vi "Disconnect.vi"(0 "reference in":refnum<class "SwitchBase.lvclass">, 1 "channel 1":string caption="Chan", 5 "error in (no error)":errorcluster) -> (14 "reference in":refnum<class "SwitchBase.lvclass">, 19 "error out":errorcluster)   [LabVIEW 2017]
uses:
  SwitchBase.lvclass
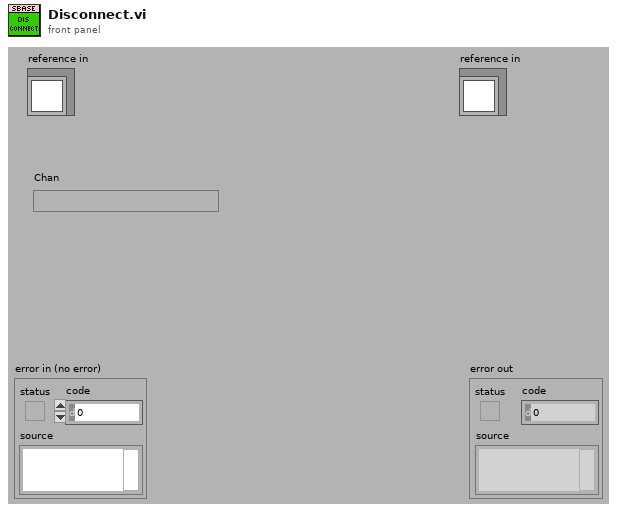
[diagram p1: front panel]
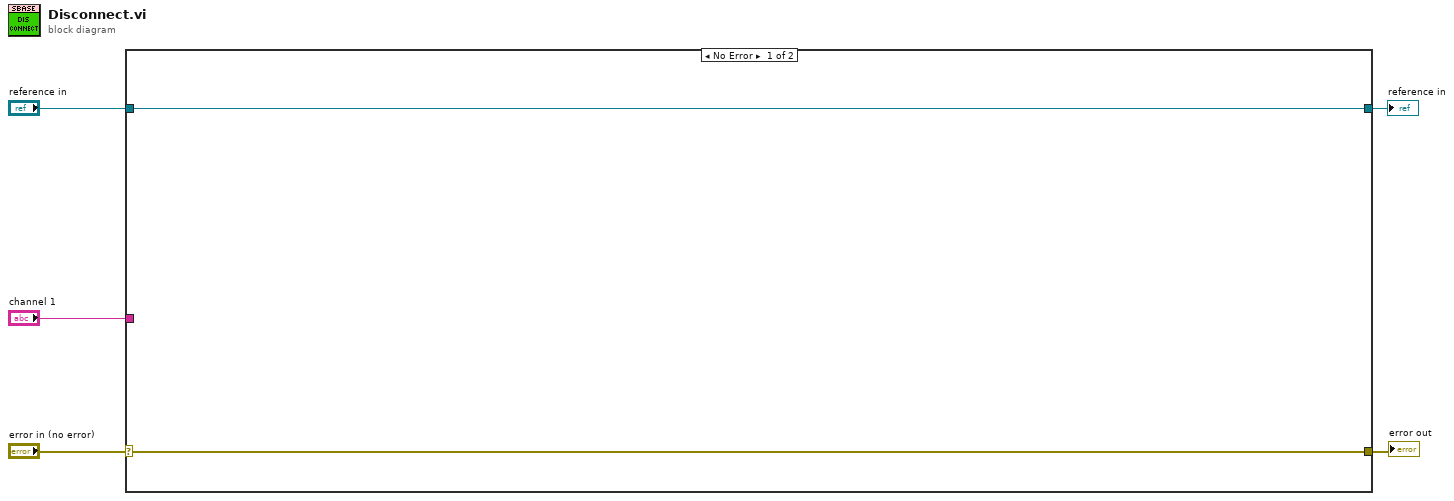
[diagram p0: block diagram]
diagram:
  n1 = case shown="No Error" "error in (no error)" {
    selector: "error in (no error)" -> [w7 w9]
    tunnel: [w7 w9] -> w4
    tunnel: [w6 w8] -> w2
    tunnel: "reference in" -> [w6 w8]
    tunnel: "channel 1" -> [_ _]
    frame No Error {
    }
    frame Error {
    }
  }
  "error out" <- w4
  "reference in" <- w2
